vi "Write (recursive).vi"(6 "ChildTag":string, 7 "Options":T1, 9 "ParentTag":string, 10 "Anything":variant, 11 "Tree in":refnum<vi>) -> (0 "error out":errorcluster, 3 "Tree out":refnum<vi>)   [LabVIEW 2019, in "BlueVariantView.lvlib"]
uses:
  BlueVariantView.lvlib
  API/Typedefs/Options.ctl
  SymbolEnumToIndex.vi
  IsErrorCluster.vi
  <vilib>/Utility/error.llb/Error Cluster From Error Code.vi
  <vilib>/Utility/Data Type/Get Numeric Information.vi
  <userlib>/_OpenG.lib/lvdata/lvdata.llb/Get Physical Units__ogtk.vi
  <vilib>/Utility/Data Type/Get Cluster Information.vi
  <vilib>/Utility/LVClass/Get LV Class Name.vi
  <vilib>/PNR/LabVIEW Composition/Composition/Decompose LabVIEW Object.vi
  <vilib>/PNR/LabVIEW Composition/Composition/Decompose Map.vi
  <userlib>/_OpenG.lib/lvdata/lvdata.llb/Array Size(s)__ogtk.vi
  <vilib>/Utility/error.llb/Trim Whitespace.vi
  <vilib>/ErrorRing/Error Ring.xnode
  <vilib>/Utility/Data Type/NI_Data Type.lvlib
  <vilib>/PNR/LabVIEW Composition/Composition/Composition.lvlib
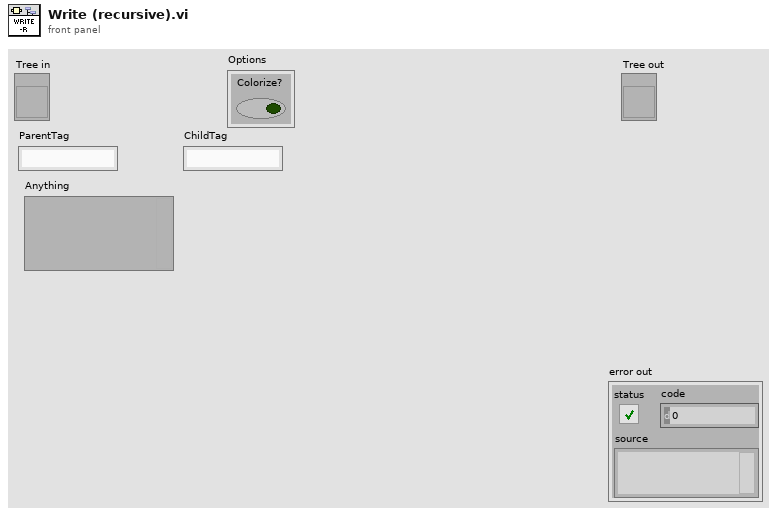
[diagram p1: front panel]
types:
  T1 = typedef "BlueVariantView.lvlib/Options.ctl" = cluster{"Colorize?":bool}
  T2 = typedef "NI_Data Type.lvlib/Data Type.ctl" = enum8{"Invalid Type", "Void", "I8", "I16", "I32", "I64", "U8", "U16", "U32", "U64", "Single Float", "Double Float", "Extended Float", "Single Complex", "Double Complex", "Extended Complex", "Enum U8", "Enum U16", "Enum U32", "Enum U64", "Single Float With Unit", "Double Float With Unit", "Extended Float With Unit", "Single Complex with Unit", "Double Complex with Unit", "Extended Complex with Unit", "Boolean", "String", "Path", "Picture", "Tag", "Array", "Cluster", "Variant", "LV Variant", "Waveform", "Timestamp", "Digital Waveform", "Digital Data", "ExpressData", "Refnum", "External Data", "VI", "Poly VI", "LabVIEW Class Instance", "Fixed Point", "Set Collection", "Map Collection"}
  T3 = typedef "BlueVariantView.lvlib/Symbol.ctl" = enum16{"None", "Cluster-brown", "Cluster-yellow", "Cluster-black", "Cluster-pink", "Array", "Float", "Int", "Bool", "String", "Enum", "Object", "Map", "Set", "Refnum", "Variant", "Path", "Picture", "Waveform", "Timestamp", "Digital Waveform", "Fixed Point"}
  T4 = typedef "BlueVariantView.lvlib/DecomposedObject.ctl" = cluster{"class name":string, "class version":string, "Private Data":variant}
  T5 = typedef "BlueVariantView.lvlib/DecomposedMap.ctl" = cluster{"Key":variant, "Value":variant}
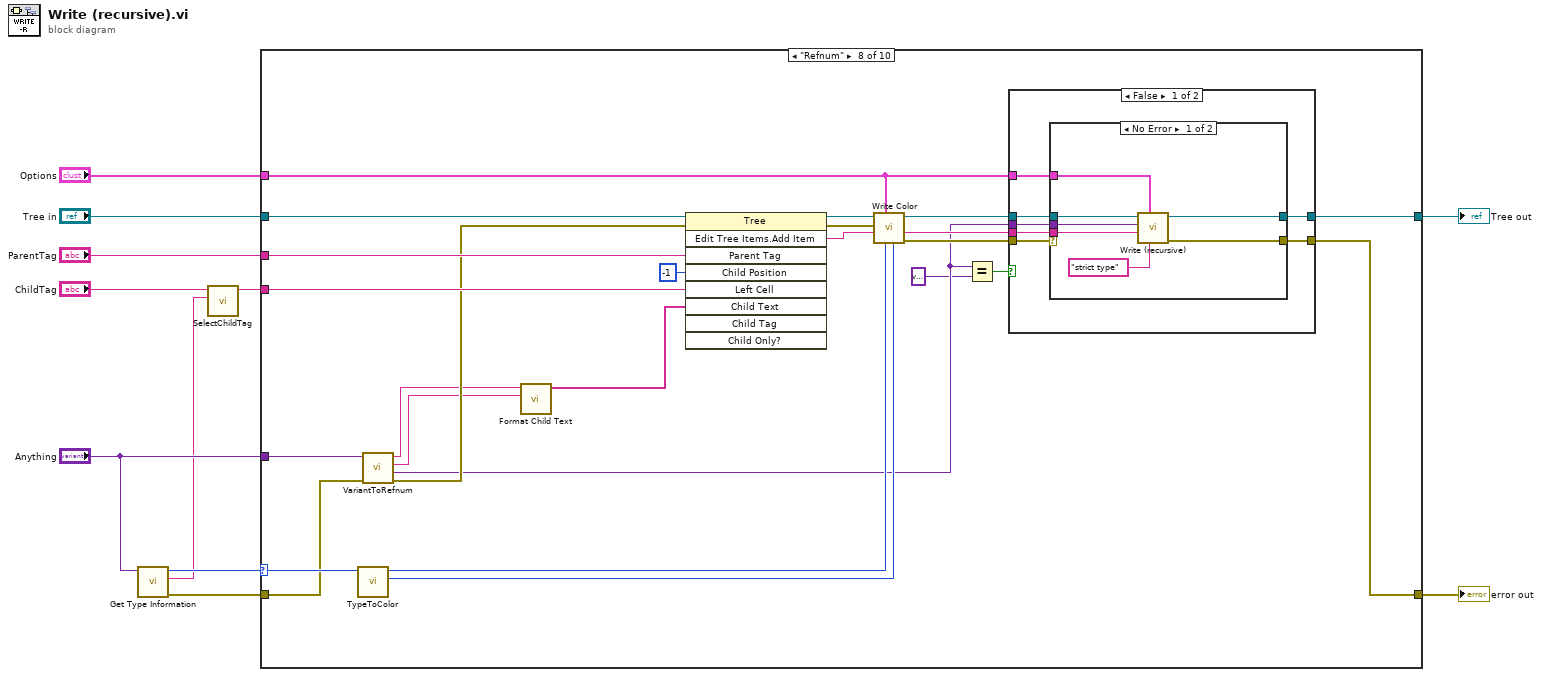
[diagram p0: block diagram]
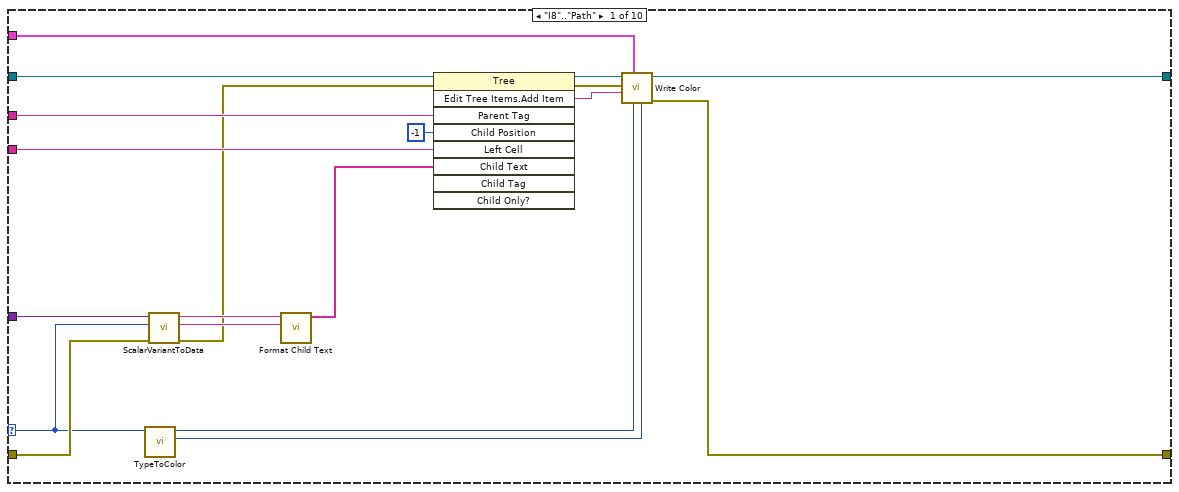
[diagram p2: hidden frame]
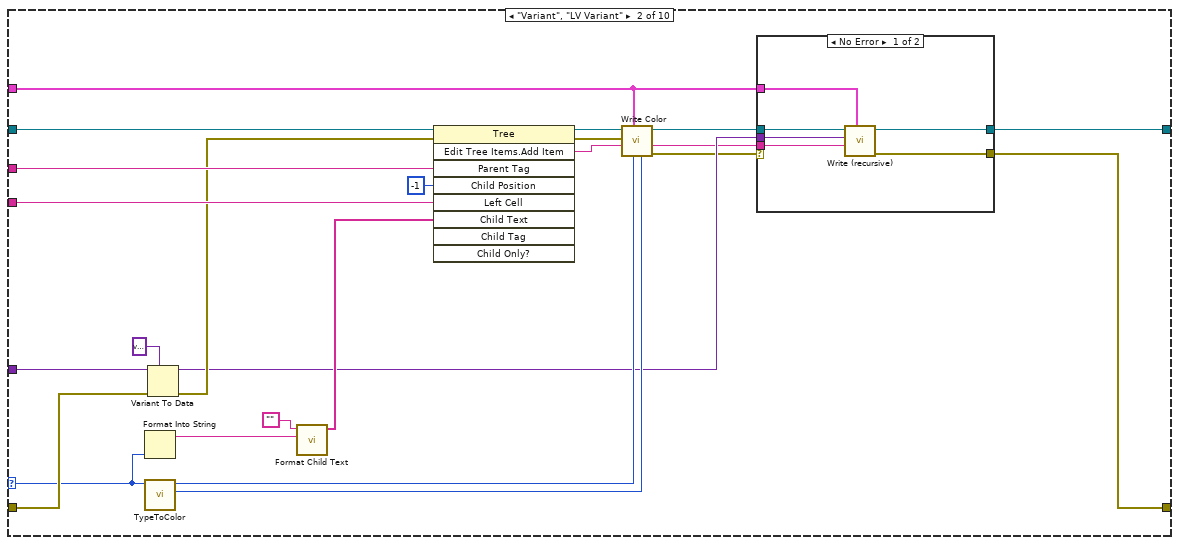
[diagram p3: hidden frame]
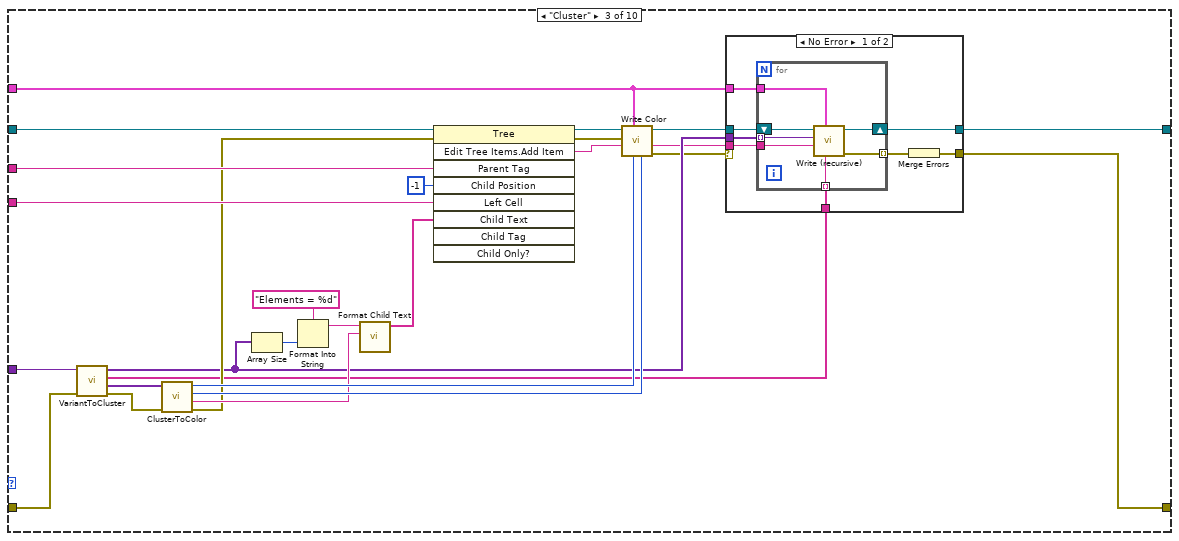
[diagram p5: hidden frame]
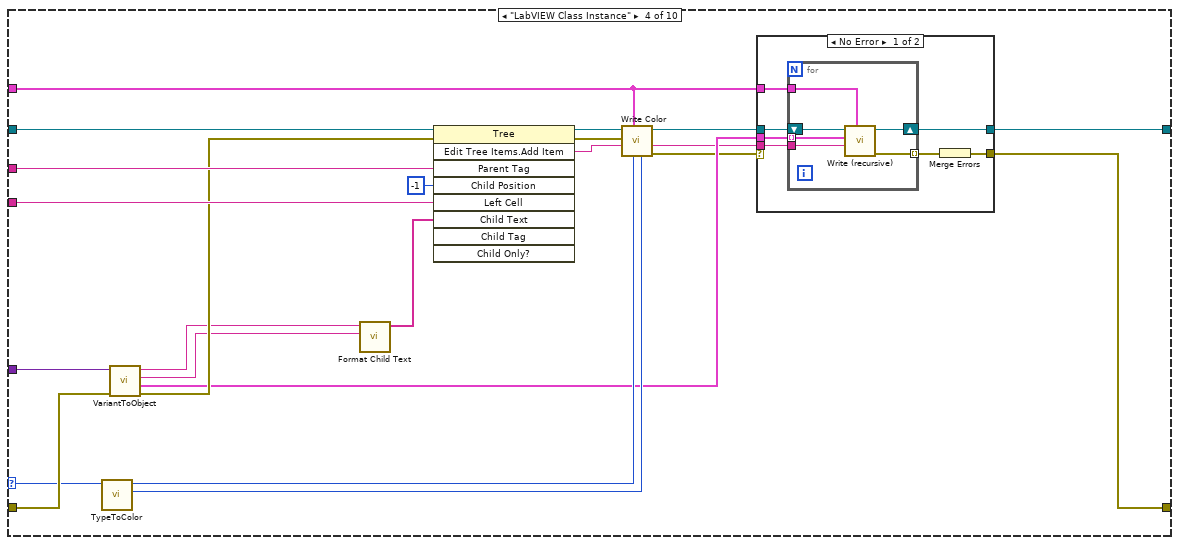
[diagram p7: hidden frame]
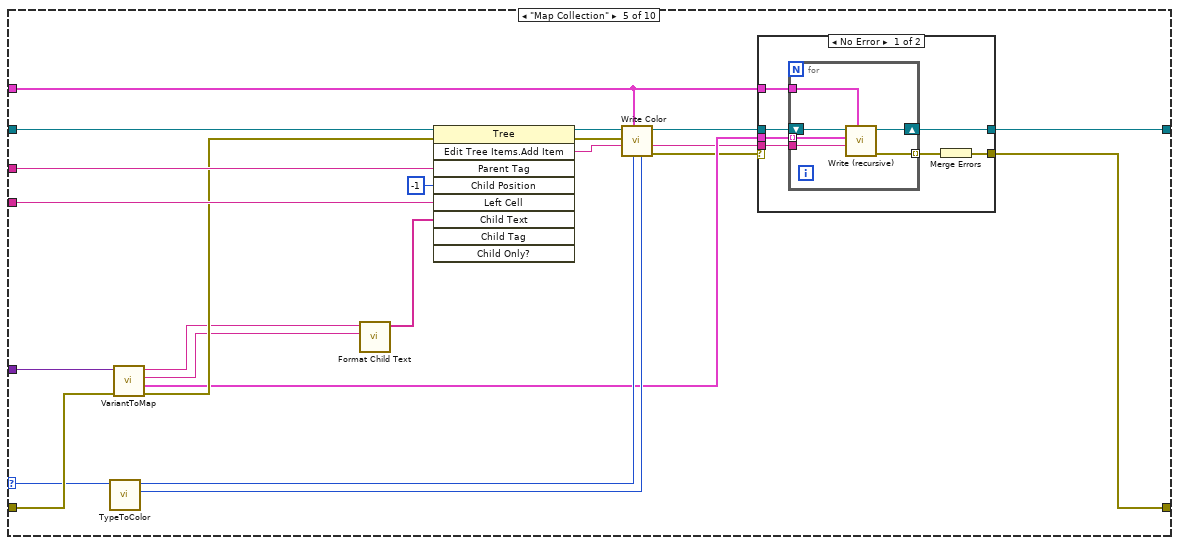
[diagram p9: hidden frame]
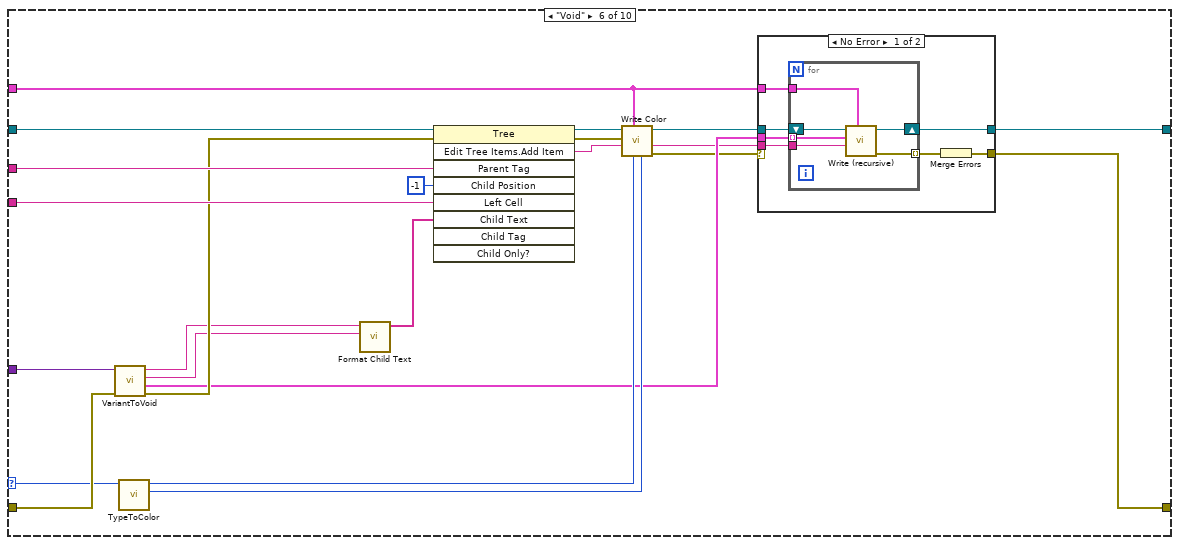
[diagram p11: hidden frame]
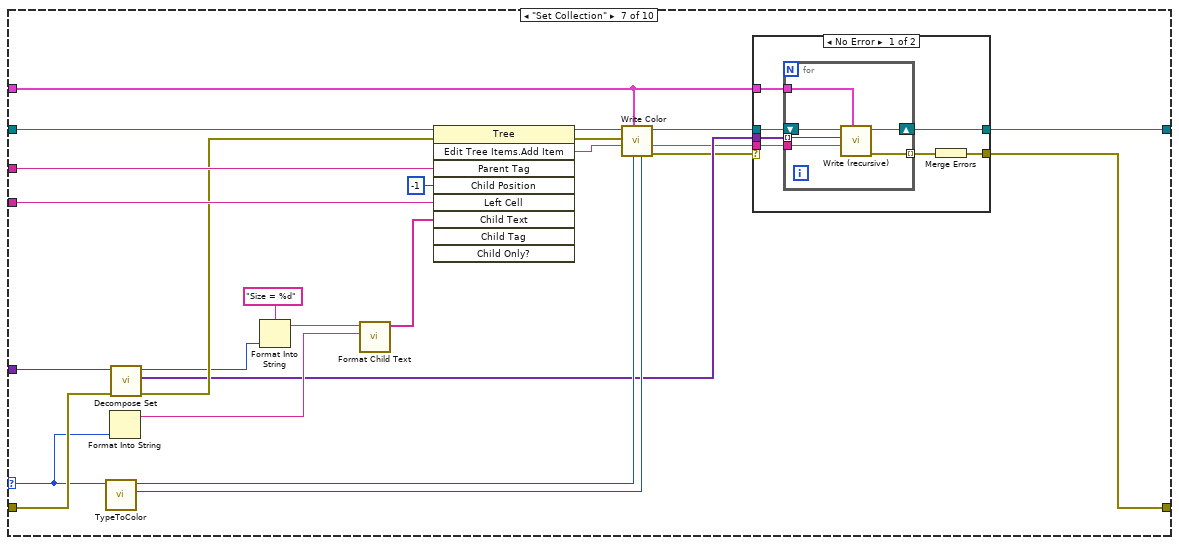
[diagram p13: hidden frame]
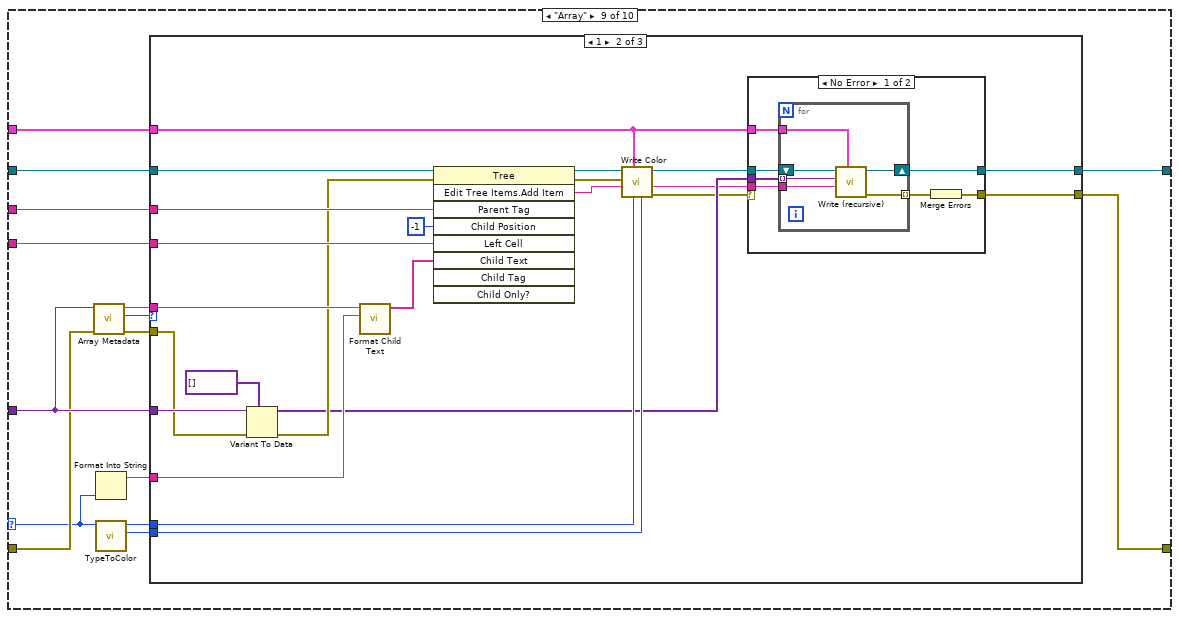
[diagram p17: hidden frame]
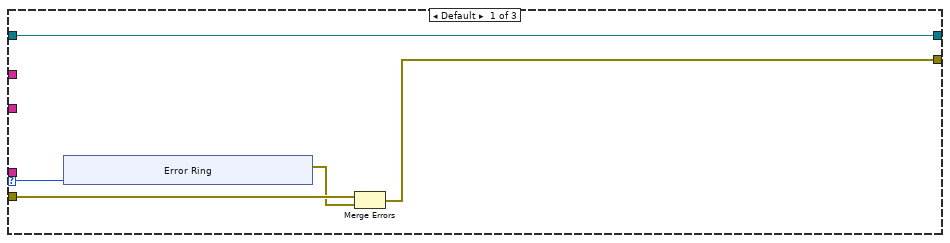
[diagram p18: hidden frame]
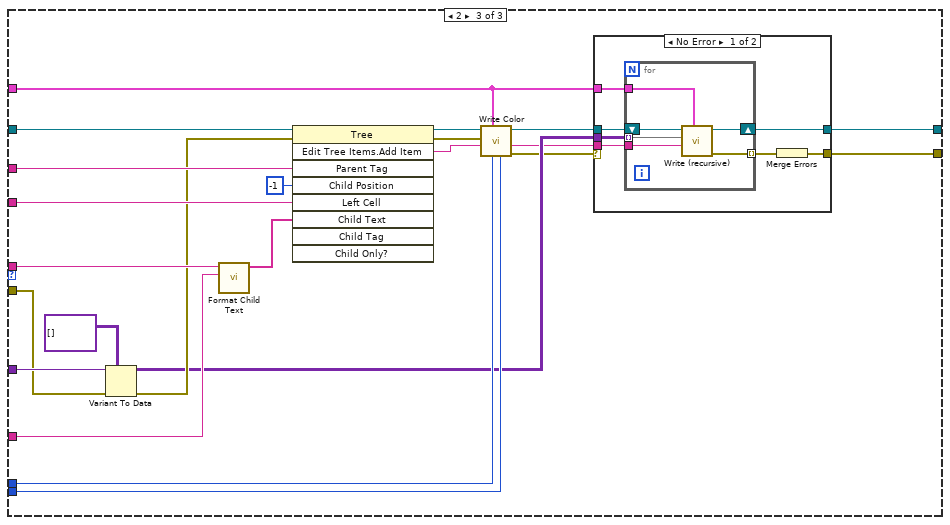
[diagram p20: hidden frame]
diagram:
  n1 = call <vilib>:"Get Type Information.vi"("variant"="Anything") -> ("error out"=w6:errorcluster, "name"=w1:string, "type"=w11:T2)  [unwired: 6 in, 2 out]
  n2 = call "SelectChildTag.vi"("Name"=w1, "ChildTag"="ChildTag") -> ("Left Cell String"=w3:string)  [unwired: 9 in]
  n3 = case shown="\"Refnum\"" w11 {
    selector: w11 -> [w15 w40 _ w116 w154 w192 w230 w272 w306 w409]
    tunnel: "Tree in" -> [w30 w54 w89 w129 w167 w205 w245 w285 w318 w426]
    tunnel: "ParentTag" -> [w29 w53 w88 w128 w166 w204 w244 w284 w317 w425]
    tunnel: "Anything" -> [w17 w52 w74 w121 w159 w197 w237 w269 w311 w419]
    tunnel: w3 -> [w26 w48 w85 w125 w163 w201 w241 w281 w315 w421]
    tunnel: [w23 w31 w66 w108 w146 w184 w222 w275 w313 w413] -> w7
    tunnel: w6 -> [w16 w47 w73 w120 w158 w196 w236 w268 w307 w418]
    tunnel: [w20 w32 w63 w107 w145 w183 w221 w261 w312 w410] -> w5
    tunnel: "Options" -> [w24 w37 w69 w113 w151 w189 w227 w276 w314 w412]
    frame "I8".."Path" {
      n4 = call "TypeToColor.vi"("type"=w15) -> ("Symbol"=w12:T3, "Color"=w13:u32)  [unwired: 9 in]
      n5 = call "ScalarVariantToData.vi"("error in (no error)"=w16, "type"=w15, "Variant"=w17) -> ("error out"=w14:errorcluster, "Type"=w18:string, "Value"=w19:string)  [unwired: 6 in]
      n6 = call "Format Child Text.vi"("Type"=w18, "Value"=w19) -> ("Child Text"=w28:string[])  [unwired: 9 in]
      n7 = invoke class="Tree" method="Edit Tree Items.Add Item"(reference=w30, error in=w14, "Parent Tag"=w29, "Child Position"=-1, "Left Cell"=w26, "Child Text"=w28) -> (reference out=w25:refnum<vi>, error out=w22:errorcluster, "Edit Tree Items:Add Item"=w21:string)  [unwired: 3 in, 6 out]
      n8 = call "Write Color.vi"("Symbol"=w12, "Color"=w13, "Options"=w24, "Tree Tag"=w21, "error in (no error)"=w22, "Tree in"=w25) -> ("error out"=w20:errorcluster, "Tree out"=w23:refnum<vi>)  [unwired: 3 in, 1 out]
    }
    frame "Variant", "LV Variant" {
      n9 = Format Into String(w40) -> (resulting string=w51:string)  [unwired: 3 in, 1 out]
      n10 = call "TypeToColor.vi"("type"=w40) -> ("Symbol"=w38:T3, "Color"=w39:u32)  [unwired: 9 in]
      n11 = Variant To Data(error in=w47, type=variant ("Anything"), Variant=w52) -> (data=w35:variant, error out=w46:errorcluster)
      n12 = call "Format Child Text.vi"("Type"=w51, "Value"="") -> ("Child Text"=w50:string[])  [unwired: 9 in]
      n13 = invoke class="Tree" method="Edit Tree Items.Add Item"(reference=w54, error in=w46, "Parent Tag"=w53, "Child Position"=-1, "Left Cell"=w48, "Child Text"=w50) -> (reference out=w45:refnum<vi>, error out=w44:errorcluster, "Edit Tree Items:Add Item"=w43:string)  [unwired: 3 in, 6 out]
      n14 = call "Write Color.vi"("Symbol"=w38, "Color"=w39, "Options"=w37, "Tree Tag"=w43, "error in (no error)"=w44, "Tree in"=w45) -> ("error out"=w33:errorcluster, "Tree Tag (dup)"=w34:string, "Tree out"=w36:refnum<vi>)  [unwired: 3 in]
      n15 = case shown="No Error" w33 {
        selector: w33 -> [_ w62]
        tunnel: w36 -> [w60 w61]
        tunnel: w37 -> [w59 _]
        tunnel: w35 -> [w58 _]
        tunnel: w34 -> [w57 _]
        tunnel: [w56 w61] -> w31
        tunnel: [w55 w62] -> w32
        frame No Error {
          n16 = call "Write (recursive).vi"("Options"=w59, "ParentTag"=w57, "Anything"=w58, "Tree in"=w60) -> ("error out"=w55:errorcluster, "Tree out"=w56:refnum<vi>)  [unwired: 6 in]
        }
        frame Error {
        }
      }
    }
    frame "Cluster" {
      n17 = call "VariantToCluster.vi"("error in (no error)"=w73, "Cluster"=w74) -> ("error out"=w72:errorcluster, "cluster elements info"=w71:variant[], "Cluster element names"=w65:string[], "Cluster elements"=w68:variant[])  [unwired: 6 in]
      n18 = call "ClusterToColor.vi"("error in (no error)"=w72, "cluster elements info"=w71) -> ("error out"=w75:errorcluster, "Type"=w76:string, "Symbol"=w77:T3, "Color"=w78:u32)  [unwired: 6 in]
      n19 = Array Size(array=w68) -> (size(s)=w81:i32)
      n20 = Format Into String(format string="Elements = %d", w81) -> (resulting string=w79:string)  [unwired: 2 in, 1 out]
      n21 = call "Format Child Text.vi"("Type"=w76, "Value"=w79) -> ("Child Text"=w87:string[])  [unwired: 9 in]
      n22 = invoke class="Tree" method="Edit Tree Items.Add Item"(reference=w89, error in=w75, "Parent Tag"=w88, "Child Position"=-1, "Left Cell"=w85, "Child Text"=w87) -> (reference out=w84:refnum<vi>, error out=w83:errorcluster, "Edit Tree Items:Add Item"=w82:string)  [unwired: 3 in, 6 out]
      n23 = call "Write Color.vi"("Symbol"=w77, "Color"=w78, "Options"=w69, "Tree Tag"=w82, "error in (no error)"=w83, "Tree in"=w84) -> ("error out"=w64:errorcluster, "Tree Tag (dup)"=w67:string, "Tree out"=w70:refnum<vi>)  [unwired: 3 in]
      n24 = case shown="No Error" w64 {
        selector: w64 -> [_ w106]
        tunnel: w70 -> [w97 w105]
        tunnel: w69 -> [w96 _]
        tunnel: w68 -> [w95 _]
        tunnel: w67 -> [w94 _]
        tunnel: [w93 w105] -> w66
        tunnel: w65 -> [w92 _]
        tunnel: [w90 w106] -> w63
        frame No Error {
          n25 = for {
            tunnel: w96 -> [w104]
            tunnel: w95 -> [w101] mode=indexing
            tunnel: w94 -> [w100]
            tunnel: w92 -> [w99] mode=indexing
            shift-right: [w102] -> w93
            shift-left: w97 -> [w103]
            tunnel: [w98] -> w91 mode=indexing
            n26 = call "Write (recursive).vi"("ChildTag"=w99, "Options"=w104, "ParentTag"=w100, "Anything"=w101, "Tree in"=w103) -> ("error out"=w98:errorcluster, "Tree out"=w102:refnum<vi>)  [unwired: 5 in]
          }
          n27 = Merge Errors(w91) -> (w90:errorcluster)
        }
        frame Error {
        }
      }
    }
    frame "LabVIEW Class Instance" {
      n28 = call "TypeToColor.vi"("type"=w116) -> ("Symbol"=w114:T3, "Color"=w115:u32)  [unwired: 9 in]
      n29 = call "VariantToObject.vi"("error in (no error)"=w120, "Object"=w121) -> ("error out"=w119:errorcluster, "DecomposedObject"=w111:T4[], "Type"=w117:string, "Value"=w118:string)  [unwired: 6 in]
      n30 = call "Format Child Text.vi"("Type"=w117, "Value"=w118) -> ("Child Text"=w127:string[])  [unwired: 9 in]
      n31 = invoke class="Tree" method="Edit Tree Items.Add Item"(reference=w129, error in=w119, "Parent Tag"=w128, "Child Position"=-1, "Left Cell"=w125, "Child Text"=w127) -> (reference out=w124:refnum<vi>, error out=w123:errorcluster, "Edit Tree Items:Add Item"=w122:string)  [unwired: 3 in, 6 out]
      n32 = call "Write Color.vi"("Symbol"=w114, "Color"=w115, "Options"=w113, "Tree Tag"=w122, "error in (no error)"=w123, "Tree in"=w124) -> ("error out"=w109:errorcluster, "Tree Tag (dup)"=w110:string, "Tree out"=w112:refnum<vi>)  [unwired: 3 in]
      n33 = case shown="No Error" w109 {
        selector: w109 -> [_ w144]
        tunnel: w112 -> [w136 w143]
        tunnel: w113 -> [w135 _]
        tunnel: w111 -> [w134 _]
        tunnel: w110 -> [w133 _]
        tunnel: [w132 w143] -> w108
        tunnel: [w130 w144] -> w107
        frame No Error {
          n34 = for {
            tunnel: w135 -> [w142]
            tunnel: w134 -> [w139] mode=indexing
            tunnel: w133 -> [w138]
            shift-right: [w140] -> w132
            shift-left: w136 -> [w141]
            tunnel: [w137] -> w131 mode=indexing
            n35 = call "Write (recursive).vi"("Options"=w142, "ParentTag"=w138, "Anything"=w139, "Tree in"=w141) -> ("error out"=w137:errorcluster, "Tree out"=w140:refnum<vi>)  [unwired: 6 in]
          }
          n36 = Merge Errors(w131) -> (w130:errorcluster)
        }
        frame Error {
        }
      }
    }
    frame "Map Collection" {
      n37 = call "TypeToColor.vi"("type"=w154) -> ("Symbol"=w152:T3, "Color"=w153:u32)  [unwired: 9 in]
      n38 = call "VariantToMap.vi"("error in (no error)"=w158, "Map"=w159) -> ("error out"=w157:errorcluster, "DecomposedMap"=w149:T5[], "Type"=w156:string, "Value"=w155:string)  [unwired: 6 in]
      n39 = call "Format Child Text.vi"("Type"=w156, "Value"=w155) -> ("Child Text"=w165:string[])  [unwired: 9 in]
      n40 = invoke class="Tree" method="Edit Tree Items.Add Item"(reference=w167, error in=w157, "Parent Tag"=w166, "Child Position"=-1, "Left Cell"=w163, "Child Text"=w165) -> (reference out=w162:refnum<vi>, error out=w161:errorcluster, "Edit Tree Items:Add Item"=w160:string)  [unwired: 3 in, 6 out]
      n41 = call "Write Color.vi"("Symbol"=w152, "Color"=w153, "Options"=w151, "Tree Tag"=w160, "error in (no error)"=w161, "Tree in"=w162) -> ("error out"=w147:errorcluster, "Tree Tag (dup)"=w148:string, "Tree out"=w150:refnum<vi>)  [unwired: 3 in]
      n42 = case shown="No Error" w147 {
        selector: w147 -> [_ w182]
        tunnel: w150 -> [w174 w181]
        tunnel: w151 -> [w173 _]
        tunnel: w149 -> [w172 _]
        tunnel: w148 -> [w171 _]
        tunnel: [w170 w181] -> w146
        tunnel: [w168 w182] -> w145
        frame No Error {
          n43 = for {
            tunnel: w173 -> [w180]
            tunnel: w172 -> [w177] mode=indexing
            tunnel: w171 -> [w176]
            shift-right: [w178] -> w170
            shift-left: w174 -> [w179]
            tunnel: [w175] -> w169 mode=indexing
            n44 = call "Write (recursive).vi"("Options"=w180, "ParentTag"=w176, "Anything"=w177, "Tree in"=w179) -> ("error out"=w175:errorcluster, "Tree out"=w178:refnum<vi>)  [unwired: 6 in]
          }
          n45 = Merge Errors(w169) -> (w168:errorcluster)
        }
        frame Error {
        }
      }
    }
    frame "Void" {
      n46 = call "VariantToVoid.vi"("error in (no error)"=w196, "Void"=w197) -> ("error out"=w195:errorcluster, "DecomposedVariant"=w187:T5[], "Type"=w193:string, "Value"=w194:string)  [unwired: 6 in]
      n47 = call "TypeToColor.vi"("type"=w192) -> ("Symbol"=w190:T3, "Color"=w191:u32)  [unwired: 9 in]
      n48 = call "Format Child Text.vi"("Type"=w193, "Value"=w194) -> ("Child Text"=w203:string[])  [unwired: 9 in]
      n49 = invoke class="Tree" method="Edit Tree Items.Add Item"(reference=w205, error in=w195, "Parent Tag"=w204, "Child Position"=-1, "Left Cell"=w201, "Child Text"=w203) -> (reference out=w200:refnum<vi>, error out=w199:errorcluster, "Edit Tree Items:Add Item"=w198:string)  [unwired: 3 in, 6 out]
      n50 = call "Write Color.vi"("Symbol"=w190, "Color"=w191, "Options"=w189, "Tree Tag"=w198, "error in (no error)"=w199, "Tree in"=w200) -> ("error out"=w185:errorcluster, "Tree Tag (dup)"=w186:string, "Tree out"=w188:refnum<vi>)  [unwired: 3 in]
      n51 = case shown="No Error" w185 {
        selector: w185 -> [_ w220]
        tunnel: w188 -> [w212 w219]
        tunnel: w189 -> [w211 _]
        tunnel: w187 -> [w210 _]
        tunnel: w186 -> [w209 _]
        tunnel: [w208 w219] -> w184
        tunnel: [w206 w220] -> w183
        frame No Error {
          n52 = for {
            tunnel: w211 -> [w218]
            tunnel: w210 -> [w215] mode=indexing
            tunnel: w209 -> [w214]
            shift-right: [w216] -> w208
            shift-left: w212 -> [w217]
            tunnel: [w213] -> w207 mode=indexing
            n53 = call "Write (recursive).vi"("Options"=w218, "ParentTag"=w214, "Anything"=w215, "Tree in"=w217) -> ("error out"=w213:errorcluster, "Tree out"=w216:refnum<vi>)  [unwired: 6 in]
          }
          n54 = Merge Errors(w207) -> (w206:errorcluster)
        }
        frame Error {
        }
      }
    }
    frame "Set Collection" {
      n55 = call "TypeToColor.vi"("type"=w230) -> ("Symbol"=w228:T3, "Color"=w229:u32)  [unwired: 9 in]
      n56 = Format Into String(w230) -> (resulting string=w232:string)  [unwired: 3 in, 1 out]
      n57 = call <vilib>:"Decompose Set.vi"("error in (no error)"=w236, "Variant"=w237) -> ("error out"=w235:errorcluster, "Elements"=w225:variant[], "Size"=w231:i32)  [unwired: 7 in]
      n58 = Format Into String(format string="Size = %d", w231) -> (resulting string=w233:string)  [unwired: 2 in, 1 out]
      n59 = call "Format Child Text.vi"("Type"=w232, "Value"=w233) -> ("Child Text"=w243:string[])  [unwired: 9 in]
      n60 = invoke class="Tree" method="Edit Tree Items.Add Item"(reference=w245, error in=w235, "Parent Tag"=w244, "Child Position"=-1, "Left Cell"=w241, "Child Text"=w243) -> (reference out=w240:refnum<vi>, error out=w239:errorcluster, "Edit Tree Items:Add Item"=w238:string)  [unwired: 3 in, 6 out]
      n61 = call "Write Color.vi"("Symbol"=w228, "Color"=w229, "Options"=w227, "Tree Tag"=w238, "error in (no error)"=w239, "Tree in"=w240) -> ("error out"=w223:errorcluster, "Tree Tag (dup)"=w224:string, "Tree out"=w226:refnum<vi>)  [unwired: 3 in]
      n62 = case shown="No Error" w223 {
        selector: w223 -> [_ w260]
        tunnel: w226 -> [w252 w259]
        tunnel: w227 -> [w251 _]
        tunnel: w225 -> [w250 _]
        tunnel: w224 -> [w249 _]
        tunnel: [w248 w259] -> w222
        tunnel: [w246 w260] -> w221
        frame No Error {
          n63 = for {
            tunnel: w251 -> [w258]
            tunnel: w250 -> [w255] mode=indexing
            tunnel: w249 -> [w254]
            shift-right: [w256] -> w248
            shift-left: w252 -> [w257]
            tunnel: [w253] -> w247 mode=indexing
            n64 = call "Write (recursive).vi"("Options"=w258, "ParentTag"=w254, "Anything"=w255, "Tree in"=w257) -> ("error out"=w253:errorcluster, "Tree out"=w256:refnum<vi>)  [unwired: 6 in]
          }
          n65 = Merge Errors(w247) -> (w246:errorcluster)
        }
        frame Error {
        }
      }
    }
    frame "Refnum" {
      n66 = call "TypeToColor.vi"("type"=w272) -> ("Symbol"=w270:T3, "Color"=w271:u32)  [unwired: 9 in]
      n67 = call "VariantToRefnum.vi"("error in (no error)"=w268, "Refnum"=w269) -> ("error out"=w267:errorcluster, "strict type"=w264:variant, "type"=w265:string, "value"=w266:string)  [unwired: 6 in]
      n68 = call "Format Child Text.vi"("Type"=w265, "Value"=w266) -> ("Child Text"=w283:string[])  [unwired: 9 in]
      n69 = invoke class="Tree" method="Edit Tree Items.Add Item"(reference=w285, error in=w267, "Parent Tag"=w284, "Child Position"=-1, "Left Cell"=w281, "Child Text"=w283) -> (reference out=w280:refnum<vi>, error out=w279:errorcluster, "Edit Tree Items:Add Item"=w278:string)  [unwired: 3 in, 6 out]
      n70 = call "Write Color.vi"("Symbol"=w270, "Color"=w271, "Options"=w276, "Tree Tag"=w278, "error in (no error)"=w279, "Tree in"=w280) -> ("error out"=w273:errorcluster, "Tree Tag (dup)"=w274:string, "Tree out"=w277:refnum<vi>)  [unwired: 3 in]
      n71 = Equal?(x=w264, y=variant ("strict type")) -> (x = y?=w262:bool)
      n72 = case shown="False" w262 {
        tunnel: w277 -> [w291 w303]
        tunnel: w276 -> [w292 _]
        tunnel: [w287 w303] -> w275
        tunnel: w274 -> [w289 _]
        tunnel: w273 -> [w288 w302]
        tunnel: [w286 w302] -> w261
        tunnel: w264 -> [w290 _]
        frame False {
          n73 = case shown="No Error" w288 {
            selector: w288 -> [_ w301]
            tunnel: w291 -> [w299 w300]
            tunnel: w292 -> [w298 _]
            tunnel: w290 -> [w297 _]
            tunnel: w289 -> [w296 _]
            tunnel: [w295 w300] -> w287
            tunnel: [w294 w301] -> w286
            frame No Error {
              n74 = call "Write (recursive).vi"("ChildTag"="strict type", "Options"=w298, "ParentTag"=w296, "Anything"=w297, "Tree in"=w299) -> ("error out"=w294:errorcluster, "Tree out"=w295:refnum<vi>)  [unwired: 5 in]
            }
            frame Error {
            }
          }
        }
        frame True {
        }
      }
    }
    frame "Array" {
      n75 = call "Array Metadata.vi"("error in (no error)"=w307, "Array"=w311) -> ("error out"=w309:errorcluster, "number of dimensions"=w308:u32, "Value"=w310:string)  [unwired: 7 in]
      n76 = Format Into String(w306) -> (resulting string=w316:string)  [unwired: 3 in, 1 out]
      n77 = call "TypeToColor.vi"("type"=w306) -> ("Symbol"=w304:T3, "Color"=w305:u32)  [unwired: 9 in]
      n78 = case shown="1" w308 {
        selector: w308 -> [w323 _ _]
        tunnel: w318 -> [w319 w353 w391]
        tunnel: w317 -> [_ w352 w390]
        tunnel: w316 -> [_ w351 w389]
        tunnel: w315 -> [_ w348 w386]
        tunnel: w305 -> [_ w339 w377]
        tunnel: w314 -> [_ w337 w375]
        tunnel: [w319 w332 w370] -> w313
        tunnel: [w320 w331 w369] -> w312
        tunnel: w311 -> [_ w343 w381]
        tunnel: w310 -> [_ w342 w380]
        tunnel: w309 -> [w322 w341 w379]
        tunnel: w304 -> [_ w338 w376]
        frame Default {
          n79 = xnode "Error Ring"("parameter 0"=w323) -> ("error out"=w321:errorcluster)
          n80 = Merge Errors(w322, w321) -> (w320:errorcluster)
        }
        frame 1 {
          n81 = Variant To Data(error in=w341, type=variant[] [], Variant=w343) -> (data=w335:variant[], error out=w340:errorcluster)
          n82 = call "Format Child Text.vi"("Type"=w351, "Value"=w342) -> ("Child Text"=w350:string[])  [unwired: 9 in]
          n83 = invoke class="Tree" method="Edit Tree Items.Add Item"(reference=w353, error in=w340, "Parent Tag"=w352, "Child Position"=-1, "Left Cell"=w348, "Child Text"=w350) -> (reference out=w347:refnum<vi>, error out=w346:errorcluster, "Edit Tree Items:Add Item"=w345:string)  [unwired: 3 in, 6 out]
          n84 = call "Write Color.vi"("Symbol"=w338, "Color"=w339, "Options"=w337, "Tree Tag"=w345, "error in (no error)"=w346, "Tree in"=w347) -> ("error out"=w333:errorcluster, "Tree Tag (dup)"=w334:string, "Tree out"=w336:refnum<vi>)  [unwired: 3 in]
          n85 = case shown="No Error" w333 {
            selector: w333 -> [_ w368]
            tunnel: w336 -> [w360 w367]
            tunnel: w337 -> [w359 _]
            tunnel: w335 -> [w358 _]
            tunnel: w334 -> [w357 _]
            tunnel: [w356 w367] -> w332
            tunnel: [w354 w368] -> w331
            frame No Error {
              n86 = for {
                tunnel: w359 -> [w366]
                tunnel: w358 -> [w363] mode=indexing
                tunnel: w357 -> [w362]
                shift-right: [w364] -> w356
                shift-left: w360 -> [w365]
                tunnel: [w361] -> w355 mode=indexing
                n87 = call "Write (recursive).vi"("Options"=w366, "ParentTag"=w362, "Anything"=w363, "Tree in"=w365) -> ("error out"=w361:errorcluster, "Tree out"=w364:refnum<vi>)  [unwired: 6 in]
              }
              n88 = Merge Errors(w355) -> (w354:errorcluster)
            }
            frame Error {
            }
          }
        }
        frame 2 {
          n89 = Variant To Data(error in=w379, type=variant[][] [], Variant=w381) -> (data=w373:variant[][], error out=w378:errorcluster)
          n90 = call "Format Child Text.vi"("Type"=w389, "Value"=w380) -> ("Child Text"=w388:string[])  [unwired: 9 in]
          n91 = invoke class="Tree" method="Edit Tree Items.Add Item"(reference=w391, error in=w378, "Parent Tag"=w390, "Child Position"=-1, "Left Cell"=w386, "Child Text"=w388) -> (reference out=w385:refnum<vi>, error out=w384:errorcluster, "Edit Tree Items:Add Item"=w383:string)  [unwired: 3 in, 6 out]
          n92 = call "Write Color.vi"("Symbol"=w376, "Color"=w377, "Options"=w375, "Tree Tag"=w383, "error in (no error)"=w384, "Tree in"=w385) -> ("error out"=w372:errorcluster, "Tree Tag (dup)"=w371:string, "Tree out"=w374:refnum<vi>)  [unwired: 3 in]
          n93 = case shown="No Error" w372 {
            selector: w372 -> [_ w406]
            tunnel: w374 -> [w398 w405]
            tunnel: w375 -> [w397 _]
            tunnel: w373 -> [w396 _]
            tunnel: w371 -> [w395 _]
            tunnel: [w394 w405] -> w370
            tunnel: [w392 w406] -> w369
            frame No Error {
              n94 = for {
                tunnel: w397 -> [w404]
                tunnel: w396 -> [w401] mode=indexing
                tunnel: w395 -> [w400]
                shift-right: [w402] -> w394
                shift-left: w398 -> [w403]
                tunnel: [w399] -> w393 mode=indexing
                n95 = call "Write (recursive).vi"("Options"=w404, "ParentTag"=w400, "Anything"=w401, "Tree in"=w403) -> ("error out"=w399:errorcluster, "Tree out"=w402:refnum<vi>)  [unwired: 6 in]
              }
              n96 = Merge Errors(w393) -> (w392:errorcluster)
            }
            frame Error {
            }
          }
        }
      }
    }
    frame Default {
      n97 = Format Into String(w409) -> (resulting string=w424:string)  [unwired: 3 in, 1 out]
      n98 = Flatten To String(anything=w419, prepend array or string size? (T)=FALSE, error in (no error)=w418) -> (data string=w417:string, error out=w416:errorcluster)  [unwired: 1 in, 1 out]
      n99 = call "TypeToColor.vi"("type"=w409) -> ("Symbol"=w407:T3, "Color"=w408:u32)  [unwired: 9 in]
      n100 = call "Format Child Text.vi"("Type"=w424, "Value"=w417) -> ("Child Text"=w423:string[])  [unwired: 9 in]
      n101 = invoke class="Tree" method="Edit Tree Items.Add Item"(reference=w426, error in=w416, "Parent Tag"=w425, "Child Position"=-1, "Left Cell"=w421, "Child Text"=w423) -> (reference out=w415:refnum<vi>, error out=w414:errorcluster, "Edit Tree Items:Add Item"=w411:string)  [unwired: 3 in, 6 out]
      n102 = call "Write Color.vi"("Symbol"=w407, "Color"=w408, "Options"=w412, "Tree Tag"=w411, "error in (no error)"=w414, "Tree in"=w415) -> ("error out"=w410:errorcluster, "Tree out"=w413:refnum<vi>)  [unwired: 3 in, 1 out]
    }
  }
  "error out" <- w5
  "Tree out" <- w7
